vi "register.vi"() -> ()   [LabVIEW 2014]
uses:
  <vilib>/registry/registry.llb/Registry RtKey.ctl
  <vilib>/registry/registry.llb/Registry SAM.ctl
  <vilib>/registry/registry.llb/Read Registry Value Simple STR.vi
  <vilib>/registry/registry.llb/Write Registry Value Simple STR.vi
panel:
  out "注册成功":string
  in  "注册":bool
  in  "请输入序列号":string
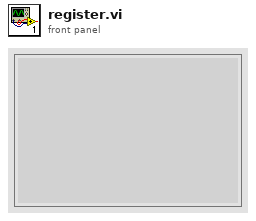
[diagram p1: front panel]
types:
  T1 = typedef "Registry SAM.ctl" = enum32{"KEY_QUERY_VALUE", "KEY_SET_VALUE", "KEY_CREATE_SUB_KEY", "KEY_ENUMERATE_SUB_KEYS", "KEY_NOTIFY", "KEY_CREATE_LINK", "KEY_READ", "KEY_WRITE", "KEY_ALL_ACCESS", "KEY_READ | KEY_WRITE"}
  T2 = typedef "Registry RtKey.ctl" = enum32{"HKEY_CLASSES_ROOT", "HKEY_CURRENT_USER", "HKEY_LOCAL_MACHINE", "HKEY_USERS", "HKEY_PERFORMANCE_DATA", "HKEY_CURRENT_CONFIG", "HKEY_DYN_DATA"}
  T3 = typedef "Registry refnum.ctl" = refnum<k1>
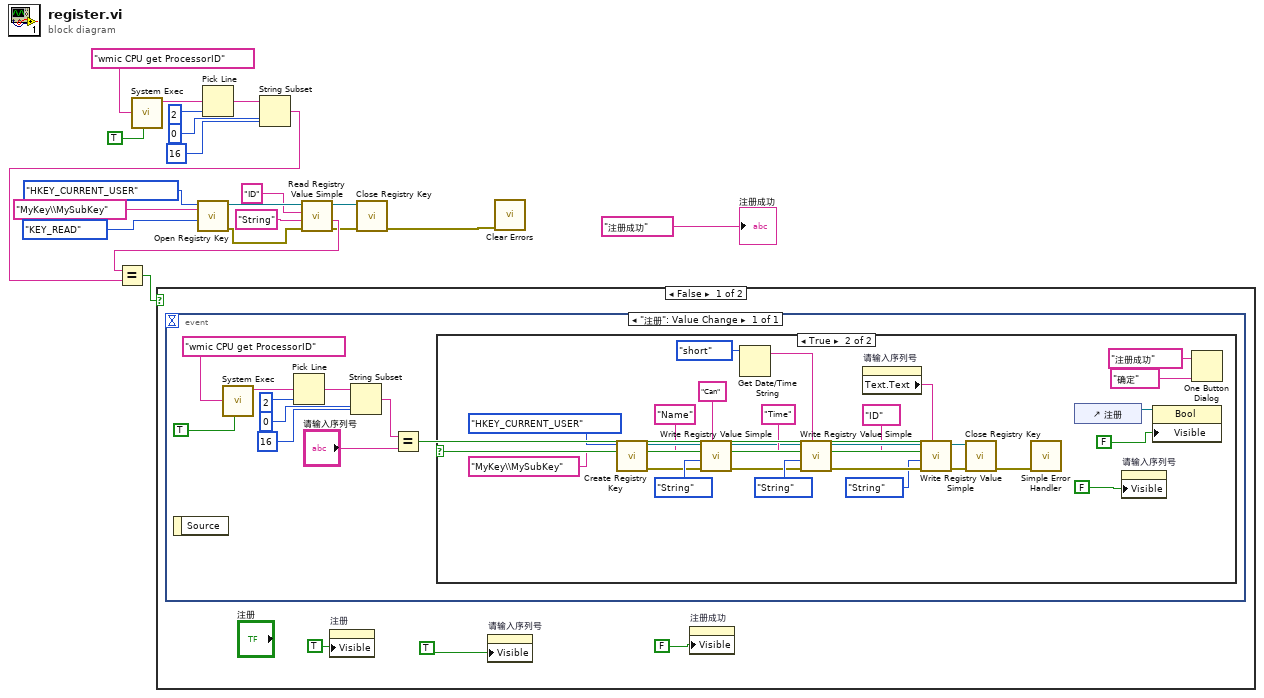
[diagram p0: block diagram]
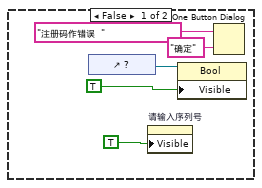
[diagram p2: hidden frame]
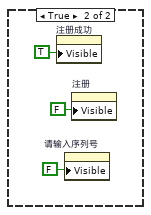
[diagram p3: hidden frame]
diagram:
  n1 = call <vilib>:"System Exec.vi"("run minimized? (F)"=TRUE, "command line"="wmic CPU get ProcessorID") -> ("standard output"=w6:string)  [unwired: 6 in, 3 out]
  n2 = call <vilib>:"Open Registry Key.vi"("security access mask (KEY_READ | KEY_WRITE)"=Registry_SAM."KEY_READ", "subkey"="MyKey\\MySubKey", "root key (HKEY_LOCAL_MACHINE)"=Registry_RtKey."HKEY_CURRENT_USER") -> ("error out"=w12:errorcluster, "refnum out"=w18:T3)  [unwired: 7 in]
  n3 = Pick Line(multi-line string=w6, line index=2) -> (output string=w8:string)  [unwired: 1 in]
  n4 = String Subset(string=w8, offset (0)=0 ("偏移量(0)"), length (rest)=16 ("长度（剩余）")) -> (substring=w3:string)
  n5 = call-poly <vilib>:"Read Registry Value Simple.vi"("error in (no error)"=w12, "default data"="String", "value"="ID", "refnum"=w18) -> ("error out"=w13:errorcluster, "String/Binary data"=w15:string, "refnum out"=w17:T3)  [unwired: 2 in, 1 out]
  n6 = Equal?(x=w15, y=w3) -> (x = y?=w14:bool)
  n7 = case shown="False" w14 {
    frame False {
      n8 = event shown="[0] \"注册\": Value Change" {
        selector: _ -> [_]
        dyn-events: _ -> [_]
        timeout: _ -> [_]
        event "注册": Value Change {
          n9 = event-data ("事件数据节点")() -> ()  [unwired: 1 in, 1 out]
          n10 = call <vilib>:"System Exec.vi"("run minimized? (F)"=TRUE, "command line"="wmic CPU get ProcessorID") -> ("standard output"=w27:string)  [unwired: 6 in, 3 out]
          n11 = Pick Line(multi-line string=w27, line index=2) -> (output string=w29:string)  [unwired: 1 in]
          n12 = String Subset(string=w29, offset (0)=0 ("偏移量(0)"), length (rest)=16 ("长度（剩余）")) -> (substring=w32:string)
          n13 = Equal?(x=w32, y="请输入序列号") -> (x = y?=w34:bool)
          n14 = case shown="True" w34 {
            frame False {
              n15 = control-ref of="?"() -> (w36:refnum<vi>)
              n16 = property on="请输入序列号" class="Str"("Visible"=TRUE ("可见")) -> ()  [unwired: 2 in, 2 out]
              n17 = property on="属性节点" class="Bool"(reference=w36, "Visible"=TRUE ("可见")) -> ()  [unwired: 1 in, 2 out]
              n18 = One Button Dialog(message="注册码作错误  " ("消息"), button name ("OK")="确定" ("按钮名称（“确定”）")) -> ()  [unwired: 1 out]
            }
            frame True {
              n19 = call <vilib>:"Create Registry Key.vi"("subkey"="MyKey\\MySubKey", "root key (HKEY_LOCAL_MACHINE)"=Registry_RtKey."HKEY_CURRENT_USER") -> ("error out"=w54:errorcluster, "refnum out"=w58:T3)  [unwired: 7 in, 1 out]
              n20 = call-poly <vilib>:"Write Registry Value Simple.vi"("String/Binary data"="Can" ("String"), "error in (no error)"=w54, "simple data type"=enum16{"String", "Binary", "DWORD"}."String", "value"="Name", "refnum"=w58) -> ("error out"=w49:errorcluster, "refnum out"=w50:T3)  [unwired: 3 in]
              n21 = Get Date/Time String(date format (0)=enum16{"short", "long", "abbreviated"}."short" ("日期格式(0)")) -> (date string=w47:string)  [unwired: 2 in, 1 out]
              n22 = call-poly <vilib>:"Write Registry Value Simple.vi"("String/Binary data"=w47, "error in (no error)"=w49, "simple data type"=enum16{"String", "Binary", "DWORD"}."String", "value"="Time", "refnum"=w50) -> ("error out"=w44:errorcluster, "refnum out"=w46:T3)  [unwired: 3 in]
              n23 = property on="请输入序列号" class="Str"() -> ("Text.Text"=w40:string)  [unwired: 2 in, 2 out]
              n24 = call-poly <vilib>:"Write Registry Value Simple.vi"("String/Binary data"=w40, "error in (no error)"=w44, "simple data type"=enum16{"String", "Binary", "DWORD"}."String", "value"="ID", "refnum"=w46) -> ("error out"=w42:errorcluster, "refnum out"=w41:T3)  [unwired: 3 in]
              n25 = call <vilib>:"Close Registry Key.vi"("error in (no error)"=w42, "refnum"=w41) -> ("error out"=w59:errorcluster)  [unwired: 5 in]
              n26 = call <vilib>:"Simple Error Handler.vi"("error in (no error)"=w59) -> ()  [unwired: 4 in, 5 out]
              n27 = control-ref of="注册"() -> (w62:refnum<vi>)
              n28 = property on="请输入序列号" class="Str"("Visible"=FALSE ("可见")) -> ()  [unwired: 2 in, 2 out]
              n29 = property on="属性节点" class="Bool"(reference=w62, "Visible"=FALSE ("可见")) -> ()  [unwired: 1 in, 2 out]
              n30 = One Button Dialog(message="注册成功" ("消息"), button name ("OK")="确定" ("按钮名称（“确定”）")) -> ()  [unwired: 1 out]
            }
          }
        }
      }
      n31 = property on="注册" class="Bool"("Visible"=TRUE ("可见")) -> ()  [unwired: 2 in, 2 out]
      n32 = property on="请输入序列号" class="Str"("Visible"=TRUE ("可见")) -> ()  [unwired: 2 in, 2 out]
      n33 = property on="注册成功" class="Str"("Visible"=FALSE ("可见")) -> ()  [unwired: 2 in, 2 out]
    }
    frame True {
      n34 = property on="注册成功" class="Str"("Visible"=TRUE ("可见")) -> ()  [unwired: 2 in, 2 out]
      n35 = property on="请输入序列号" class="Str"("Visible"=FALSE ("可见")) -> ()  [unwired: 2 in, 2 out]
      n36 = property on="注册" class="Bool"("Visible"=FALSE ("可见")) -> ()  [unwired: 2 in, 2 out]
    }
  }
  n37 = call <vilib>:"Close Registry Key.vi"("error in (no error)"=w13, "refnum"=w17) -> ("error out"=w1:errorcluster)  [unwired: 5 in]
  n38 = call <vilib>:"Clear Errors.vi"("error in (no error)"=w1) -> ()  [unwired: 5 in, 2 out]
  "注册成功" <- "注册成功"
